vi "Move.vi"(0 "handle":u32, 1 "Distance":sgl, 2 "Decel":sgl, 3 "Move Method":i32, 4 "Direct of movement":i32, 5 "Axis":i32, 7 "Sramp":sgl, 9 "Accel":sgl, 11 "error in (no error)":errorcluster caption="错误输入（无错误）", 12 "Lspeed":sgl, 13 "Speed":sgl, 14 "Move Mode":i32) -> (15 "error out":errorcluster caption="错误输出")   [LabVIEW 2015]
uses:
  zauxdll-2014/zauxdll.lvlib
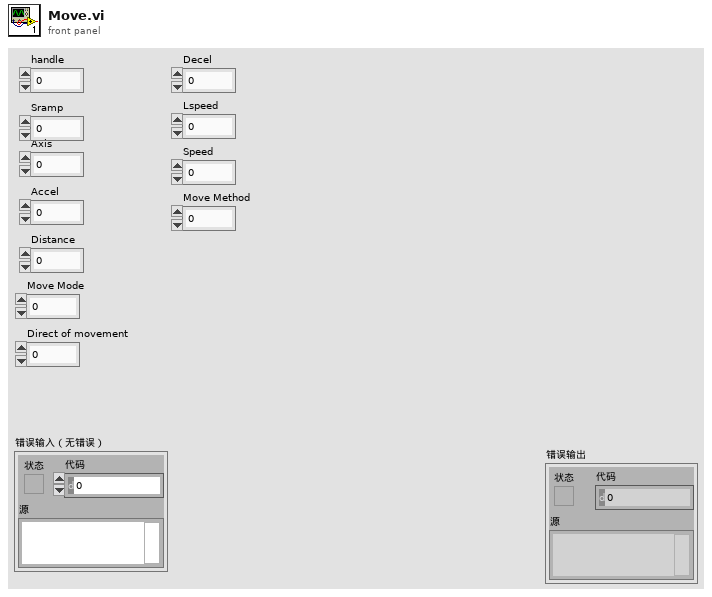
[diagram p1: front panel]
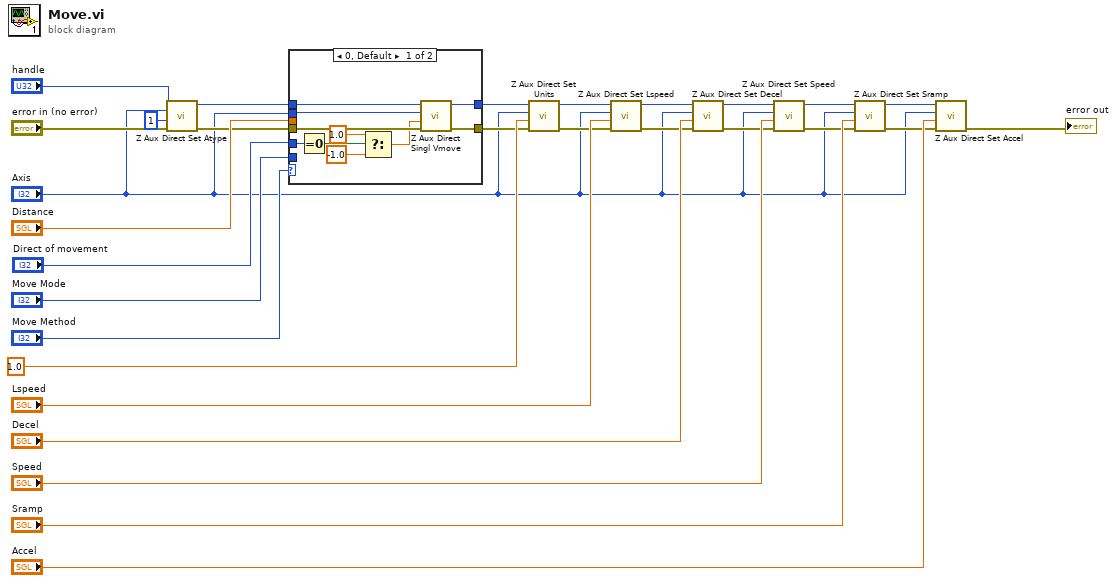
[diagram p0: block diagram]
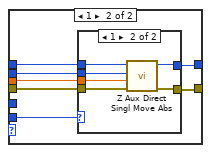
[diagram p2: hidden frame]
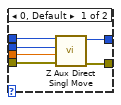
[diagram p3: hidden frame]
diagram:
  n1 = call "Z Aux Direct Set Atype.vi"("error in (no error)"="error in (no error)", "iValue"=1, "iaxis"="Axis", "handle"="handle") -> ("error out"=w14:errorcluster, "handle out"=w28:u32)  [unwired: 5 in, 1 out]
  n2 = case shown="0, Default" "Move Method" {
    tunnel: w28 -> [w39 w45]
    tunnel: [w38 w43] -> w27
    tunnel: "Distance" -> [_ w40]
    tunnel: w14 -> [w37 w46]
    tunnel: [w36 w44] -> w13
    tunnel: "Axis" -> [w35 w41]
    tunnel: "Move Mode" -> [_ w42]
    tunnel: "Direct of movement" -> [w34 _]
    frame 0, Default {
      n3 = Equal To 0?(x=w34) -> (x = 0?=w33:bool)
      n4 = Select(t=1.0, s=w33, f=-1.0) -> (s? t:f=w30:dbl)
      n5 = call "Z Aux Direct Singl Vmove.vi"("error in (no error)"=w37, "idir"=w30, "iaxis"=w35, "handle"=w39) -> ("error out"=w36:errorcluster, "handle out"=w38:u32)  [unwired: 5 in, 1 out]
    }
    frame 1 {
      n6 = case shown="1" w42 {
        tunnel: w46 -> [w52 w56]
        tunnel: w45 -> [w51 w58]
        tunnel: [w50 w55] -> w44
        tunnel: [w49 w57] -> w43
        tunnel: w41 -> [w48 w54]
        tunnel: w40 -> [w47 w53]
        frame 0, Default {
          n7 = call "Z Aux Direct Singl Move.vi"("error in (no error)"=w52, "fdistance"=w47, "iaxis"=w48, "handle"=w51) -> ("error out"=w50:errorcluster, "handle out"=w49:u32)  [unwired: 5 in, 1 out]
        }
        frame 1 {
          n8 = call "Z Aux Direct Singl Move Abs.vi"("error in (no error)"=w56, "fdistance"=w53, "iaxis"=w54, "handle"=w58) -> ("error out"=w55:errorcluster, "handle out"=w57:u32)  [unwired: 5 in, 1 out]
        }
      }
    }
  }
  n9 = call "Z Aux Direct Set Units.vi"("error in (no error)"=w13, "fValue"=sgl 1.0 ("Units"), "iaxis"="Axis", "handle"=w27) -> ("error out"=w8:errorcluster, "handle out"=w9:u32)  [unwired: 5 in, 1 out]
  n10 = call "Z Aux Direct Set Lspeed.vi"("error in (no error)"=w8, "fValue"="Lspeed", "iaxis"="Axis", "handle"=w9) -> ("error out"=w7:errorcluster, "handle out"=w6:u32)  [unwired: 5 in, 1 out]
  n11 = call "Z Aux Direct Set Decel.vi"("error in (no error)"=w7, "fValue"="Decel", "iaxis"="Axis", "handle"=w6) -> ("error out"=w12:errorcluster, "handle out"=w26:u32)  [unwired: 5 in, 1 out]
  n12 = call "Z Aux Direct Set Speed.vi"("error in (no error)"=w12, "fValue"="Speed", "iaxis"="Axis", "handle"=w26) -> ("error out"=w11:errorcluster, "handle out"=w25:u32)  [unwired: 5 in, 1 out]
  n13 = call "Z Aux Direct Set Sramp.vi"("error in (no error)"=w11, "fValue"="Sramp", "iaxis"="Axis", "handle"=w25) -> ("error out"=w10:errorcluster, "handle out"=w24:u32)  [unwired: 5 in, 1 out]
  n14 = call "Z Aux Direct Set Accel.vi"("error in (no error)"=w10, "fValue"="Accel", "iaxis"="Axis", "handle"=w24) -> ("error out"=→"error out":errorcluster)  [unwired: 5 in, 2 out]
